vi "Connect Channels.vi"   [LabVIEW 2020, in "SLSC Switch.lvlib"]
doc: "Creates connections between channels."
uses:
  <vilib>/SLSC_Switch/SLSC Switch.lvlib
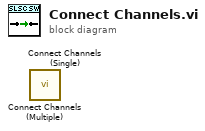
[diagram p0: block diagram]
diagram:
  n1 = call <vilib>:"Connect Channels (Multiple).vi"() -> ()  [unwired: 10 in, 2 out]
  n2 = call <vilib>:"Connect Channels (Single).vi"() -> ()  [unwired: 10 in, 2 out]
